vi "x in range absolute value 3 and half.vi"(1 "Numeric":fxp<+/-,20,5> format="%.17g") -> (0 "y":fxp<+/-,20,5> format="%.17g")   [LabVIEW 2009]
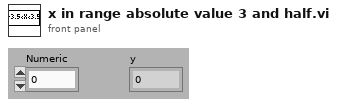
[diagram p1: front panel]
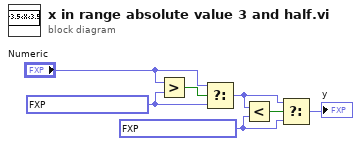
[diagram p0: block diagram]
diagram:
  w6 = fxp<+/-,20,5> 3.5 ("y")
  w3 = fxp<+/-,20,5> -3.5 ("y")
  n1 = Greater?(x="Numeric", y=w3) -> (0:w2:bool)
  n2 = Select(t="Numeric", s=w2, f=w3) -> (s? t:f=w1:fxp<+/-,20,5>)
  n3 = Less?(x=w1, y=w6) -> (x < y?=w4:bool)
  n4 = Select(t=w1, s=w4, f=w6) -> (s? t:f=→"y":fxp<+/-,20,5>)
